vi "dfd_Multirate Filter Design Param Transfer.vi"(6 "option":enum16{"Normal", "Nyquist", "Alias free"}(ring), 7 "multirate factor":i32=4, 8 "error in (no error)":errorcluster, 10 "roll off":dbl format="%.2f", 11 "order":i32) -> (0 "error out":errorcluster, 1 "fstop":dbl, 2 "fpass":dbl, 3 "new order":i32)   [LabVIEW 2017, in "NI_DigFilterLicensed.lvlib"]
uses:
  <vilib>/addons/Digital Filter Design/NI_DigFilterLicensed.lvlib
  <vilib>/addons/Digital Filter Design/_Misc.llb/dfd_Error Handlers (Single).vi
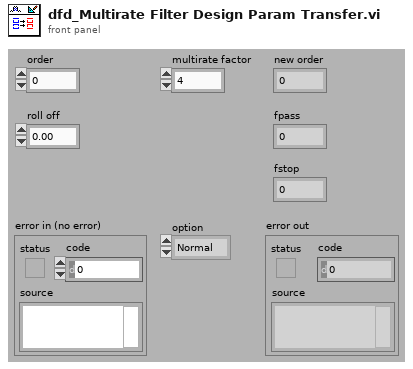
[diagram p1: front panel]
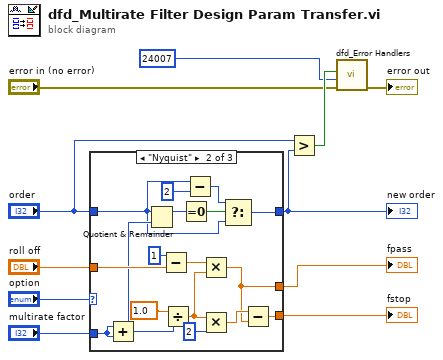
[diagram p0: block diagram]
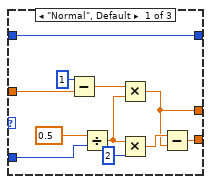
[diagram p2: hidden frame]
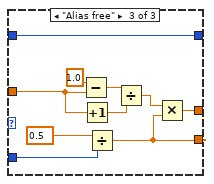
[diagram p3: hidden frame]
diagram:
  n1 = case shown="\"Nyquist\"" "option" {
    tunnel: "roll off" -> [w21 w39 w45]
    tunnel: "multirate factor" -> [w22 w30 w44]
    tunnel: [w14 w32 w43] -> w8
    tunnel: [w15 w33 w42] -> w7
    tunnel: "order" -> [w12 w25 w40]
    tunnel: [w12 w23 w40] -> w6
    frame "Normal", Default {
      n2 = Subtract(x=1, y=w21) -> (x-y=w19:dbl)
      n3 = Divide(x=0.5, y=w22) -> (x/y=w18:dbl)
      n4 = Multiply(x=w19, y=w18) -> (x*y=w14:dbl)
      n5 = Multiply(x=w18, y=2) -> (x*y=w16:dbl)
      n6 = Subtract(x=w16, y=w14) -> (x-y=w15:dbl)
    }
    frame "Nyquist" {
      n7 = Add(x=w30, y=w30) -> (x+y=w29:i32)
      n8 = Quotient & Remainder(x=w25, y=w29) -> (x-y*floor(x/y)=w28:i32)  [unwired: 1 out]
      n9 = Subtract(x=1, y=w39) -> (x-y=w37:dbl)
      n10 = Divide(x=1.0, y=w29) -> (x/y=w36:dbl)
      n11 = Equal To 0?(x=w28) -> (x = 0?=w27:bool)
      n12 = Subtract(x=w25, y=2) -> (x-y=w26:i32)
      n13 = Multiply(x=w37, y=w36) -> (x*y=w32:dbl)
      n14 = Multiply(x=w36, y=2) -> (x*y=w34:dbl)
      n15 = Select(t=w26, s=w27, f=w25) -> (s? t:f=w23:i32)
      n16 = Subtract(x=w34, y=w32) -> (x-y=w33:dbl)
    }
    frame "Alias free" {
      n17 = Subtract(x=1.0, y=w45) -> (x-y=w48:dbl)
      n18 = Increment(x=w45) -> (x+1=w47:dbl)
      n19 = Divide(x=0.5, y=w44) -> (x/y=w42:dbl)
      n20 = Divide(x=w48, y=w47) -> (x/y=w46:dbl)
      n21 = Multiply(x=w46, y=w42) -> (x*y=w43:dbl)
    }
  }
  "fpass" <- w8
  "fstop" <- w7
  "new order" <- w6
  n22 = Greater?(x="order", y=w6) -> (0:w4:bool)
  n23 = call-poly <vilib>:"dfd_Error Handlers.vi"("error in (no error)"="error in (no error)", "error code"=24007 ("WRN_ZERO_COEF_REMOVED"), "condition failed?"=w4) -> ("error out"=→"error out":errorcluster)  [unwired: 8 out]
